vi "Inspect OF.vi"(11 "strout":string) -> (0 "error out":errorcluster, 2 "cas faux":string, 3 "Boolean":bool)   [LabVIEW 2020]
uses:
  <vilib>/regexp/Match Regular Expression.xnode
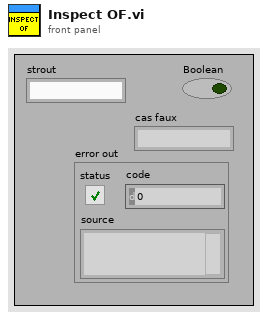
[diagram p1: front panel]
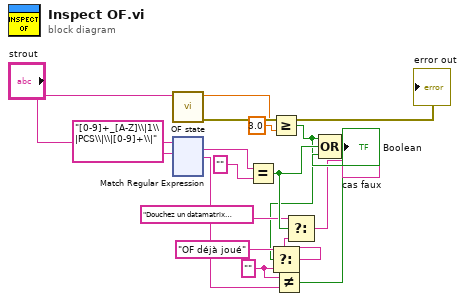
[diagram p0: block diagram]
diagram:
  w13 = "" ("cas faux")
  n1 = call "OF state.vi"("OF"="strout") -> ("error out"=→"error out":errorcluster, "number dbl"=w2:dbl)  [unwired: 8 in, 1 out]
  n2 = xnode "Match Regular Expression"("chaîne en entrée"="strout", "expression régulière"="[0-9]+_[A-Z]\\|1\\|PCS\\|\\|[0-9]+\\|") -> ("toute l'expression"=w11:string, "après la correspondance"=w14:string)  [unwired: 4 in, 3 out]
  n3 = Equal? ("Égaux ?")(x=w11, y="" ("cas faux")) -> (x = y?=w10:bool)
  n4 = Greater Or Equal? ("Supérieur ou égal ?")(x=w2, y=3.0) -> (x >= y?=w4:bool)
  n5 = Select ("Sélectionner")(t="OF déjà joué", s=w4, f=w13) -> (s? t:f=w7:string)
  n6 = Not Equal?(x=w13, y=w14) -> (x != y?=w15:bool)
  n7 = Select(t="Douchez un datamatrix correct!", s=w10, f=w7) -> (s? t:f=→"cas faux":string)
  n8 = Compound Arithmetic op=OR ("Opérateur arithmétique")(w4, w10, w15) -> (→"Boolean":bool)
